vi "in_1d interp prepare arrays.vi"(6 "ntimes":i32=1, 8 "X is monotonic":bool, 9 "xi":dbl[](array[numeric]), 10 "Y":dbl[](array[numeric]), 11 "X":dbl[](array[numeric])) -> (0 "error":i32, 1 "xi-out":dbl[](array[numeric]), 2 "Y-out":dbl[](array[numeric]), 3 "X-out":dbl[](array[numeric]), 4 "ntimes remaining":i32=1)   [LabVIEW 2017, in "NI_Gmath.lvlib"]
uses:
  NI_Gmath.lvlib
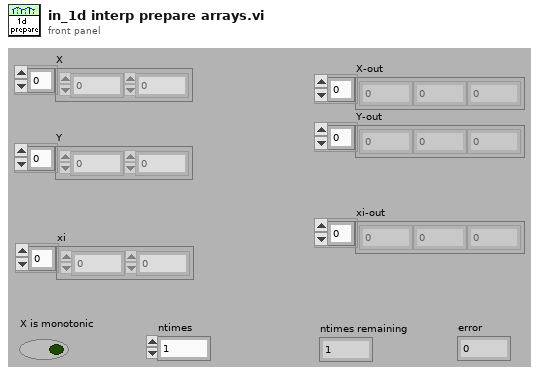
[diagram p1: front panel]
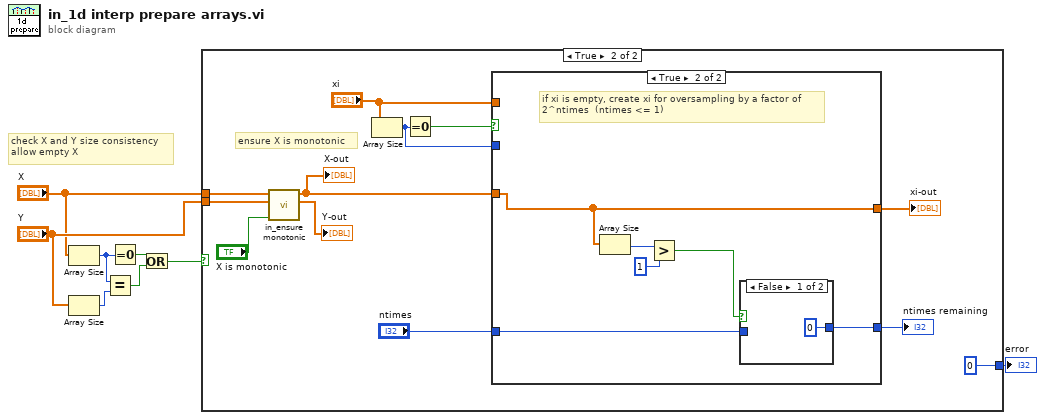
[diagram p0: block diagram]
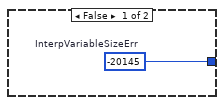
[diagram p2: hidden frame]
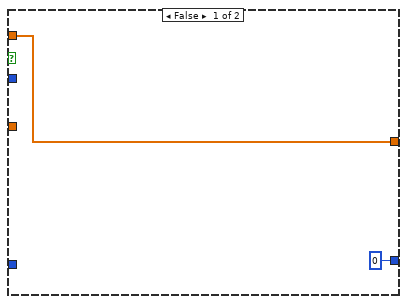
[diagram p3: hidden frame]
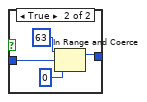
[diagram p4: hidden frame]
diagram:
  # "check X and Y size consistency\nallow empty X"
  n1 = Array Size(array="X") -> (size(s)=w4:i32)
  n2 = Array Size(array="Y") -> (size(s)=w6:i32)
  n3 = Equal?(x=w4, y=w6) -> (x = y?=w2:bool)
  n4 = Equal To 0?(x=w4) -> (x = 0?=w3:bool)
  n5 = Or(x=w3, y=w2) -> (x .or. y?=w1:bool)
  n6 = case shown="True" w1 {
    tunnel: "Y" -> [_ w12]
    tunnel: "X" -> [_ w11]
    tunnel: [w9 0 ("InterpVariableSizeErr")] -> w5
    frame False {
      w9 = -20145  # InterpVariableSizeErr
    }
    frame True {
      # "ensure X is monotonic"
      n7 = call "in_ensure monotonic.vi"("X is monotonic"="X is monotonic", "Y"=w12, "X"=w11) -> ("Y out"=→"Y-out":dbl[], "X out"=w17:dbl[])  [unwired: 7 in]
      "X-out" <- w17
      n8 = Array Size(array="xi") -> (size(s)=w21:i32)
      n9 = Equal To 0?(x=w21) -> (x = 0?=w15:bool)
      n10 = case shown="True" w15 {
        tunnel: w17 -> [_ w27]
        tunnel: [w23 w27] -> w20
        tunnel: w21 -> [_ _]
        tunnel: "xi" -> [w23 _]
        tunnel: "ntimes" -> [_ w28]
        tunnel: [0 ("upper limit") w29] -> w13
        frame False {
        }
        frame True {
          # "if xi is empty, create xi for oversampling by a factor of\n2^ntimes  (ntimes <= 1)"
          n11 = Array Size(array=w27) -> (size(s)=w26:i32)
          n12 = Greater?(x=w26, y=1 ("upper limit")) -> (0:w24:bool)
          n13 = case shown="False" w24 {
            tunnel: [0 ("upper limit") w32] -> w29
            tunnel: w28 -> [_ w31]
            frame False {
            }
            frame True {
              n14 = In Range and Coerce(upper limit=63, x=w31, lower limit=0 ("upper limit")) -> (coerced(x)=w32:i32)  [unwired: 1 out]
            }
          }
        }
      }
      "xi-out" <- w20
      "ntimes remaining" <- w13
    }
  }
  "error" <- w5
